vi "Set Max.vi"(0 "Level in":refnum<class "Level.lvclass">, 7 "Max":dbl, 9 "mod corr (dB)":dbl, 11 "error in (no error)":errorcluster) -> (4 "Level out":refnum<class "Level.lvclass">, 15 "error out":errorcluster)   [LabVIEW 2020, in "Level.lvclass"]
uses:
  Level.lvclass
  Level.lvclass/Level.ctl
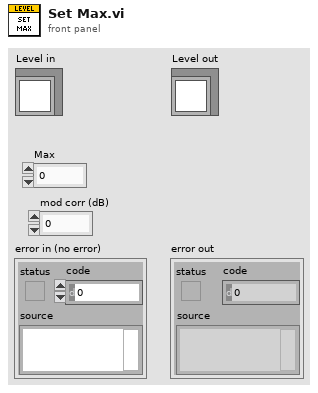
[diagram p1: front panel]
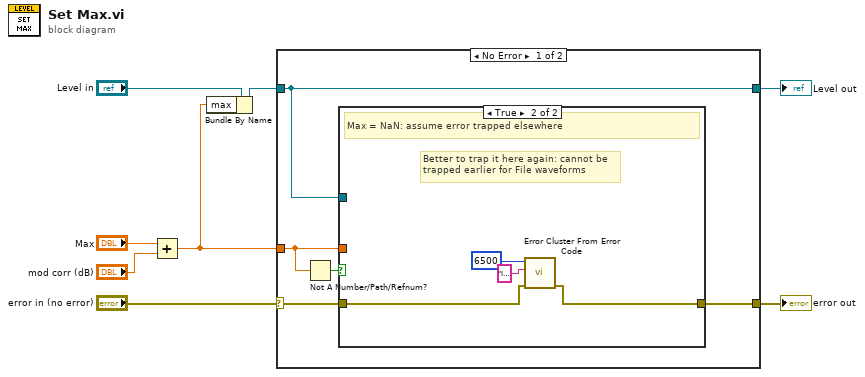
[diagram p0: block diagram]
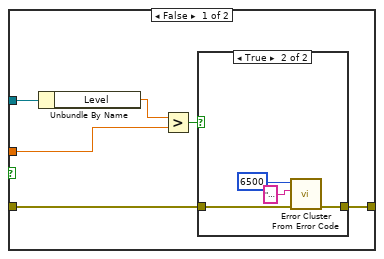
[diagram p2: hidden frame]
diagram:
  n1 = Add(x="Max", y="mod corr (dB)") -> (x+y=w2:dbl)
  n2 = Bundle By Name(cluster="Level in", "max"=w2) -> (w4:refnum<class "Level.lvclass">)
  n3 = case shown="No Error" "error in (no error)" {
    selector: "error in (no error)" -> [w10 w30]
    tunnel: [w9 w30] -> w7
    tunnel: [w13 w29] -> w5
    tunnel: w4 -> [w13 w29]
    tunnel: w2 -> [w12 _]
    frame No Error {
      n4 = Not A Number/Path/Refnum?(number/path/refnum=w12) -> (NaN/Path/Refnum?=w11:bool)
      n5 = case shown="True" w11 {
        tunnel: w12 -> [w18 _]
        tunnel: [w16 w25] -> w9
        tunnel: w10 -> [w15 w26]
        tunnel: w13 -> [w19 _]
        frame False {
          n6 = Unbundle By Name(w19) -> ("Level"=w14:dbl)
          n7 = Greater?(x=w14, y=w18) -> (0:w17:bool)
          n8 = case shown="True" w17 {
            tunnel: [w20 w23] -> w16
            tunnel: w15 -> [w20 w24]
            frame False {
            }
            frame True {
              n9 = call <vilib>:"Error Cluster From Error Code.vi"("error in (no error)"=w24, "error message (\"\")"="Level requested is greater than the max.", "error code (0)"=6500) -> ("error out"=w23:errorcluster)  [unwired: 6 in]
            }
          }
        }
        frame True {
          # "Better to trap it here again: cannot be\ntrapped earlier for File waveforms"
          # "Max = NaN: assume error trapped elsewhere"
          n10 = call <vilib>:"Error Cluster From Error Code.vi"("error in (no error)"=w26, "error message (\"\")"="Invalid level reference. If using a .wav or .f64 file, double-check that you supplied a reference.", "error code (0)"=6500) -> ("error out"=w25:errorcluster)  [unwired: 6 in]
        }
      }
    }
    frame Error {
    }
  }
  "error out" <- w7
  "Level out" <- w5
